vi "control2contraste.vi"(0 "Sound Device IN":T3 {"task ID" format="%.0x"}, 1 "Camera Device IN":T5, 2 "Image Device IN":cluster{"Image":T4, "errorImage":errorcluster}, 4 "Sound Parameters":cluster{"# samples":u32, "tiempos (ms)":dbl}, 5 "Parametros Interferometro/Freq-Volt":T6, 6 "sound?":bool, 7 "ControlSignal":dbl[](array[numeric]), 8 "Streeam?":bool, 10 "Mostrar?":bool) -> (13 "Contraste":dbl, 14 "Sound Device OUT":T3 {"task ID" format="%.0x"}, 15 "Camara Device OUT":T5, 16 "Image Device OUT":cluster{"Image":T4, "errorImage":errorcluster}, 17 "Waveform":waveform(dbl))   [LabVIEW 2010]
uses:
  <vilib>/vision/Image Controls.llb/IMAQ Image.ctl
  <vilib>/sound2/lvsound2.llb/Sound Output Task ID.ctl
  <vilib>/sound2/lvsound2.llb/Sound Data Format.ctl
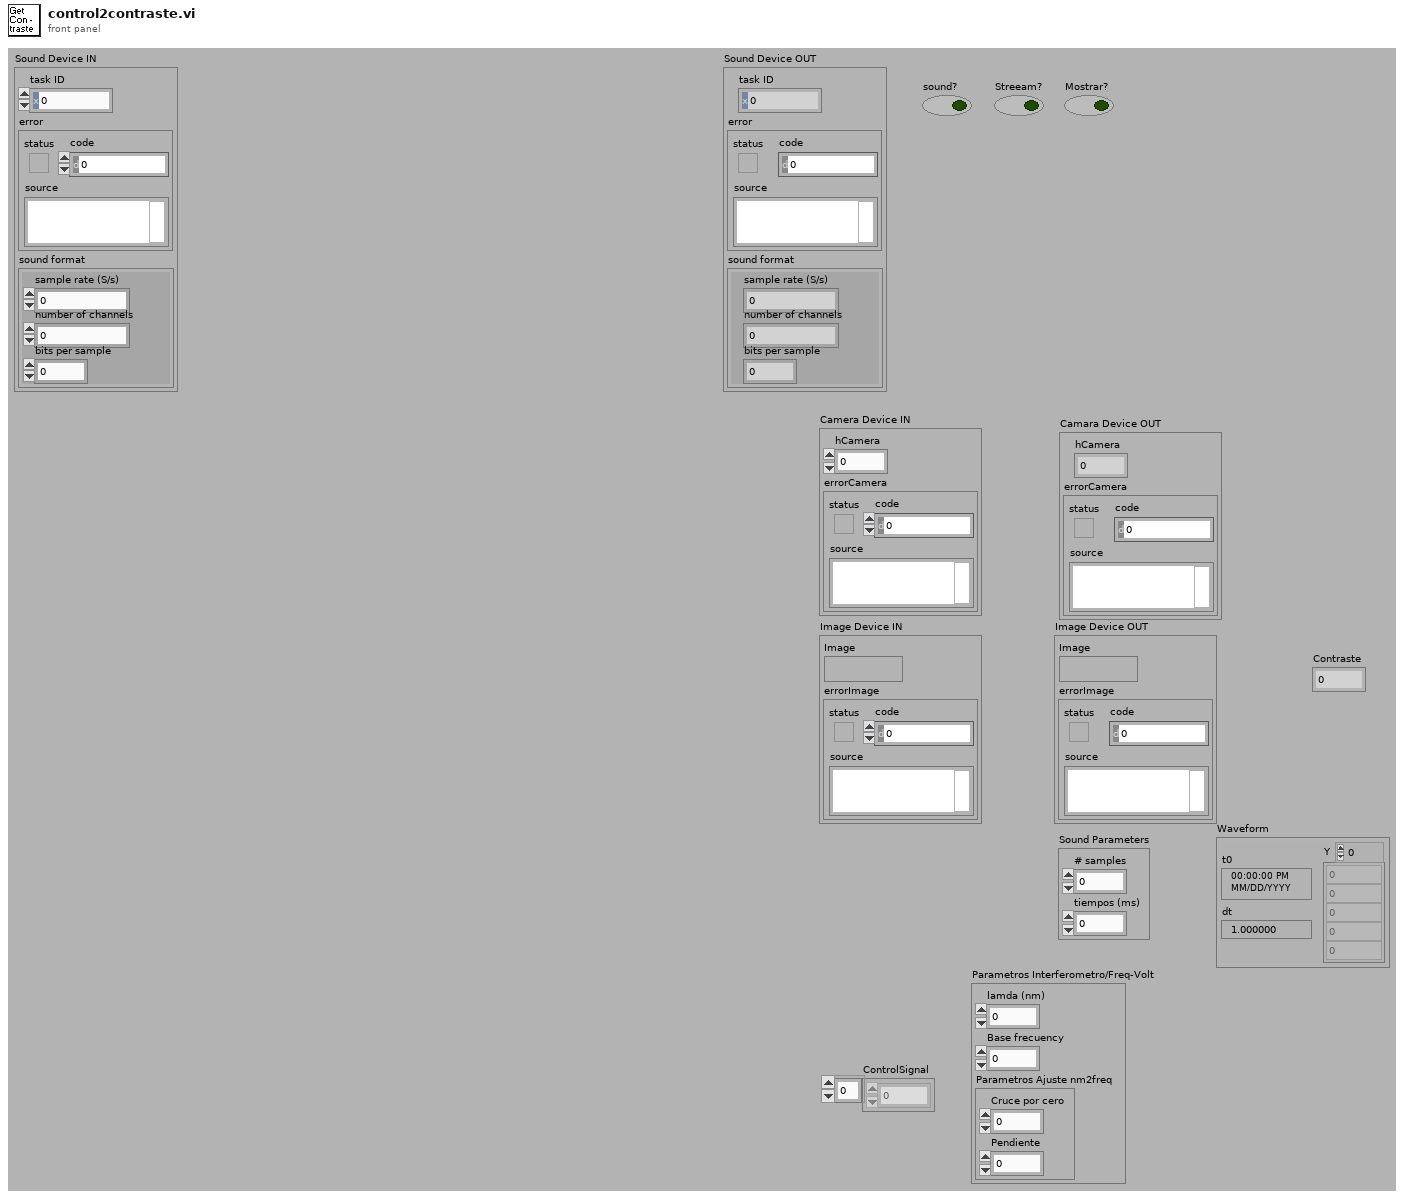
[diagram p1: front panel]
types:
  T1 = typedef "Sound Output Task ID.ctl" = u32
  T2 = typedef "Sound Data Format.ctl" = cluster{"sample rate (S/s)":dbl, "number of channels":i32, "bits per sample":i32}
  T3 = cluster{"task ID":T1, "error":errorcluster, "sound format":T2}
  T4 = typedef "IMAQ Image.ctl" = refnum<image>
  T5 = cluster{"hCamera":u32, "errorCamera":errorcluster}
  T6 = cluster{"lamda (nm)":dbl, "Base frecuency":dbl, "Parametros Ajuste nm2freq":cluster{"Cruce por cero":dbl, "Pendiente":dbl}}
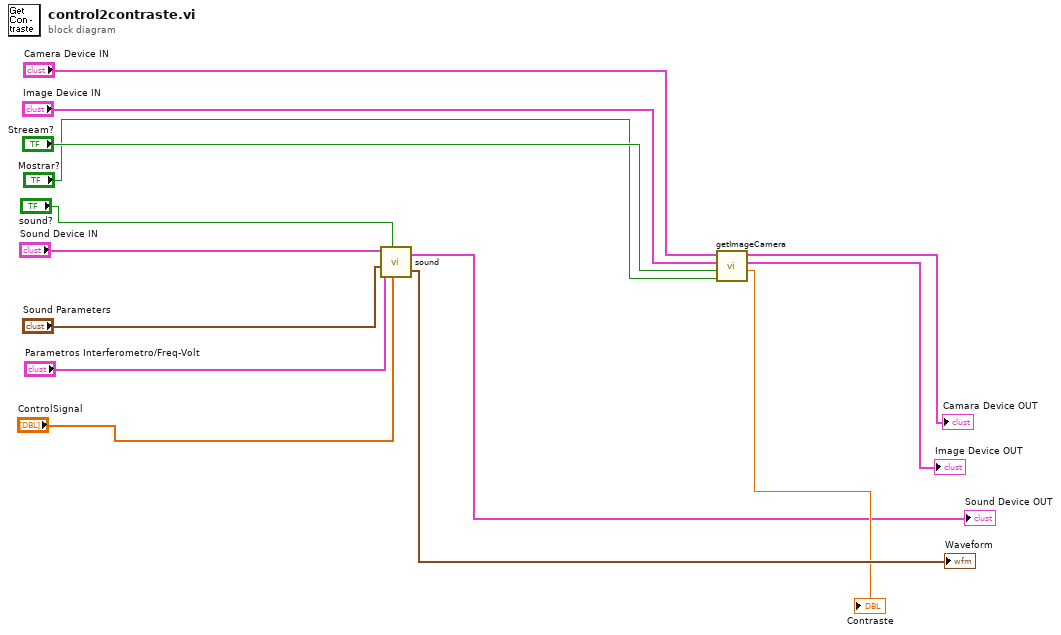
[diagram p0: block diagram]
diagram:
  n1 = call "sound.vi"("df Array"="ControlSignal", "sound?"="sound?", "Parametros Interferometro/Freq-Volt"="Parametros Interferometro/Freq-Volt", "Sound Parameters"="Sound Parameters", "Sound Device IN"="Sound Device IN") -> ("Waveform"=→"Waveform":waveform(dbl), "Sound Device OUT"=→"Sound Device OUT":T3)  [unwired: 1 in]
  n2 = call "getImageCamera.vi"("Mostrar?"="Mostrar?", "Streeam?"="Streeam?", "Image Device IN"="Image Device IN", "Camera Device IN"="Camera Device IN") -> ("Contraste OUT"=→"Contraste":dbl, "Image Device OUT"=→"Image Device OUT":cluster{"Image":T4, "errorImage":errorcluster}, "Camara Device OUT"=→"Camara Device OUT":T5)  [unwired: 1 in]
